vi "Get Parameter Value - Array of Booleans.vi"(7 "Default value":bool[](array[boolean]), 8 "error in (no error)":errorcluster, 9 "Parameter name":string, 10 "Config name":string, 11 "Config in":refnum<class "Config.lvclass">) -> (0 "error out":errorcluster, 2 "Value":bool[](array[boolean]), 3 "Config out":refnum<class "Config.lvclass">)   [LabVIEW 2026, in "TALOS.lvlib" / "Classes.lvlib" / "Config.lvclass"]
doc: "Get the parameter's value (string) from the specified configuration. Use the data type terminal to specify the output type."
uses:
  Config.lvclass
  <vilib>/AdvancedString/Delimited String to 1D String Array (string).vi
  <vilib>/Utility/error.llb/Trim Whitespace (string).vi
  <vilib>/Utility/error.llb/Trim Whitespace One-Sided.vi
  TALOS.lvlib
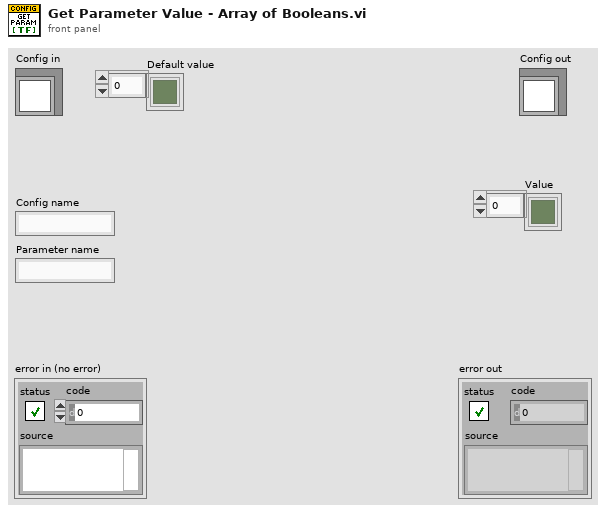
[diagram p1: front panel]
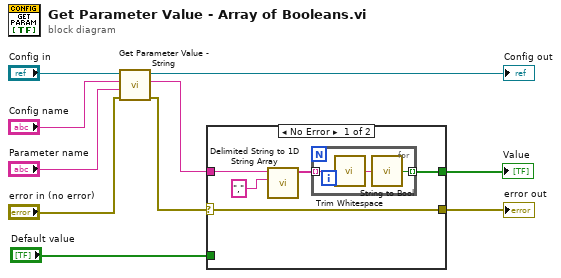
[diagram p0: block diagram]
diagram:
  n1 = call "Get Parameter Value - String.vi"("error in (no error)"="error in (no error)", "Parameter name"="Parameter name", "Config name"="Config name", "Config in"="Config in") -> ("error out"=w3:errorcluster, "Value"=w5:string, "Config out"=→"Config out":refnum<class "Config.lvclass">)  [unwired: 5 in]
  n2 = case shown="No Error" w3 {
    selector: w3 -> [w12 w19]
    tunnel: w5 -> [w15 _]
    tunnel: "Default value" -> [_ w20]
    tunnel: [w12 w19] -> w2
    tunnel: [w11 w20] -> w1
    frame No Error {
      n3 = call-poly <vilib>:"Delimited String to 1D String Array.vi"("delimiter"=",", "delimited string"=w15) -> ("string array"=w13:string[])  [unwired: 9 in]
      n4 = for {
        tunnel: w13 -> [w18] mode=indexing
        tunnel: [w16] -> w11 mode=indexing
        n5 = call-poly <vilib>:"Trim Whitespace.vi"("string"=w18) -> ("trimmed string"=w17:string)  [unwired: 1 in]
        n6 = call "String to Bool.vi"("String"=w17) -> ("Boolean"=w16:bool)
      }
    }
    frame Error {
    }
  }
  "error out" <- w2
  "Value" <- w1
